vi "类型2增加一组结果统计.vi"(8 "合格":bool, 9 "最大误差":dbl, 11 "第几组":i32) -> ()   [LabVIEW 2010]
uses:
  全局量/自动测试结果.vi
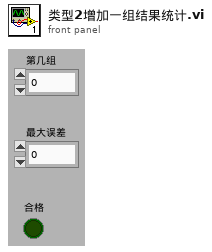
[diagram p1: front panel]
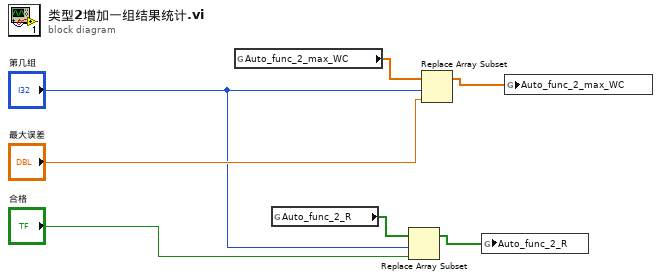
[diagram p0: block diagram]
diagram:
  n1 = global read "自动测试结果.vi" "Auto_func_2_max_WC"() -> (w7:dbl[])
  n2 = global read "自动测试结果.vi" "Auto_func_2_R"() -> (w5:bool[])
  n3 = Replace Array Subset(array=w5, new element="合格", index="第几组") -> (w1:bool[])
  n4 = Replace Array Subset(array=w7, new element="最大误差", index="第几组") -> (w2:dbl[])
  n5 = global write "自动测试结果.vi" "Auto_func_2_R"(w1) -> ()
  n6 = global write "自动测试结果.vi" "Auto_func_2_max_WC"(w2) -> ()
